vi "Create test signal for tone detection.vi"(5 "block size":i32, 6 "second tone":bool, 7 "sampling frequency (Hz)":dbl=51200.0, 9 "Noise level (Vrms)":dbl(slide) scale=0.0..10.0, 10 "Tone amplitude":dbl=0.5, 11 "Tone frequency (Hz)":dbl=2345.67) -> (3 "Test signal":waveform(dbl)(graph))   [LabVIEW 2023]
doc: "Create test signal for tone detection."
uses:
  <vilib>/Analysis/NI_AALBase.lvlib
panel:
  # "If TRUE, the second tone is 1V at 9.876 kHz."
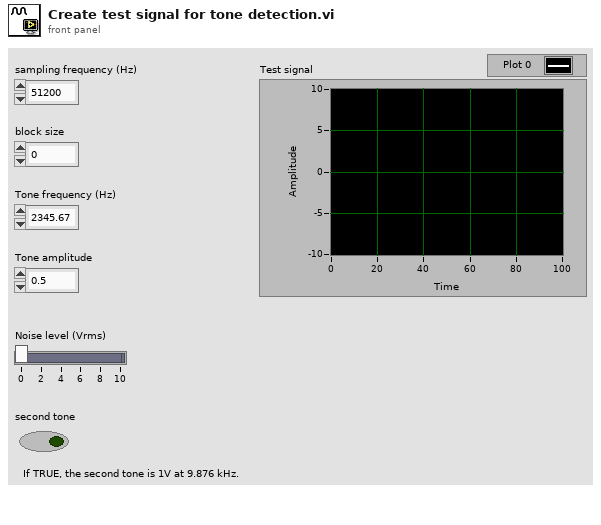
[diagram p1: front panel]
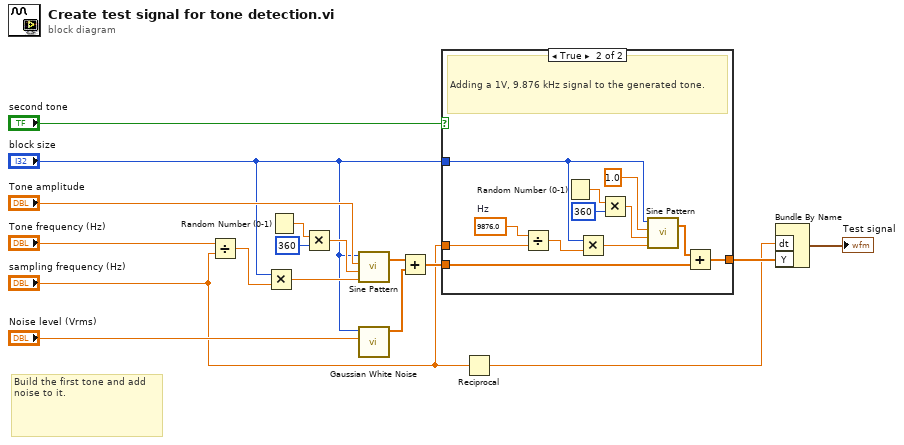
[diagram p0: block diagram]
diagram:
  # "Build the first tone and add noise to it."
  n1 = Divide(x="Tone frequency (Hz)", y="sampling frequency (Hz)") -> (x/y=w6:dbl)
  n2 = Multiply(x="block size", y=w6) -> (x*y=w12:dbl)
  n3 = Random Number (0-1)() -> (number: 0 to 1=w13:dbl)
  n4 = Multiply(x=w13, y=360) -> (x*y=w14:dbl)
  n5 = call <vilib>:"Sine Pattern.vi"("cycles"=w12, "phase(degrees)"=w14, "amplitude"="Tone amplitude", "samples"="block size") -> ("Sinusoidal Pattern"=w16:dbl[])  [unwired: 1 out]
  n6 = call <vilib>:"Gaussian White Noise.vi"("standard deviation"="Noise level (Vrms)", "samples"="block size") -> ("Gaussian noise pattern"=w17:dbl[])  [unwired: 8 in, 1 out]
  n7 = Add(x=w16, y=w17) -> (x+y=w9:dbl[])
  n8 = case shown="True" "second tone" {
    tunnel: "block size" -> [_ w26]
    tunnel: "sampling frequency (Hz)" -> [_ w25]
    tunnel: w9 -> [w18 w24]
    tunnel: [w18 w22] -> w4
    frame False {
      # "Do not add second tone."
    }
    frame True {
      w19 = 9876.0  # Hz
      # "Adding a 1V, 9.876 kHz signal to the generated tone."
      n9 = Divide(x=w19, y=w25) -> (x/y=w29:dbl)
      n10 = Random Number (0-1)() -> (number: 0 to 1=w28:dbl)
      n11 = Multiply(x=w26, y=w29) -> (x*y=w30:dbl)
      n12 = Multiply(x=w28, y=360) -> (x*y=w27:dbl)
      n13 = call <vilib>:"Sine Pattern.vi"("cycles"=w30, "phase(degrees)"=w27, "amplitude"=1.0, "samples"=w26) -> ("Sinusoidal Pattern"=w23:dbl[])  [unwired: 1 out]
      n14 = Add(x=w23, y=w24) -> (x+y=w22:dbl[])
    }
  }
  n15 = Reciprocal(x="sampling frequency (Hz)") -> (1/x=w3:dbl)
  n16 = Bundle By Name("dt"=w3, "Y"=w4) -> (→"Test signal":waveform(dbl))  [unwired: 1 in]
